vi "Tree Get Node Wild (Usage Mask).vi"(8 "error in (no error)":errorcluster, 9 "Usage mask":i32, 10 "Path":string, 11 "Tree DVR in":refnum<data-value>) -> (0 "error out":errorcluster, 2 "Node array out":refnum<data-value>, 3 "Tree DVR out":refnum<data-value>)   [LabVIEW 2012, in "MDSplus.lvlib"]
doc: "Return the TreeNode array for all the successor nodes of the specified usage with respect of the passed path."
uses:
  <vilib>/MDSplus/Library/MDSplus.lvlib
  <vilib>/MDSplus/Classes/Tree_Class/Tree.lvclass
  <vilib>/MDSplus/Classes/TreeNodeArray_Class/TreeNodeArray.lvclass
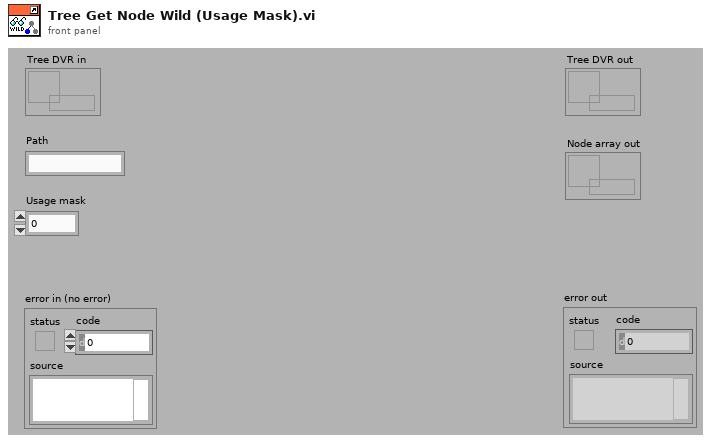
[diagram p1: front panel]
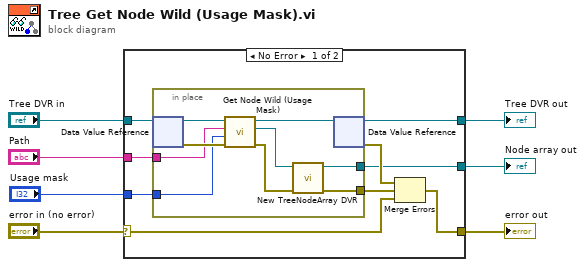
[diagram p0: block diagram]
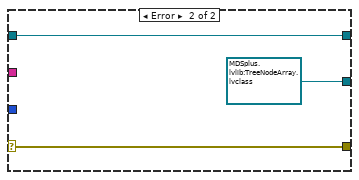
[diagram p2: hidden frame]
diagram:
  n1 = case shown="No Error" "error in (no error)" {
    selector: "error in (no error)" -> [w15 w28]
    tunnel: "Tree DVR in" -> [w16 w27]
    tunnel: [w13 w28] -> w7
    tunnel: [w12 w27] -> w4
    tunnel: [w10 refnum<data-value> refnum ("TreeNode DVR out")] -> w2
    tunnel: "Path" -> [w11 _]
    tunnel: "Usage mask" -> [w8 _]
    frame No Error {
      n2 = in-place {
        in-place-border: [w19] -> w9
        in-place-border: w11 -> [w22]
        in-place-border: [w21] -> w10
        in-place-border: w8 -> [w17]
        n3 = in-place-dvr #1(w16) -> (w25:refnum<class "Tree.lvclass">, w23:errorcluster)
        n4 = call-dynamic "Get Node Wild (Usage Mask).vi"("error in (no error)"=w23, "Usage mask"=w17, "Path"=w22, "Tree in"=w25) -> ("error out"=w20:errorcluster, "Node array out"=w18:refnum<class "TreeNodeArray.lvclass">, "Tree out"=w24:refnum<class "Tree.lvclass">)  [unwired: 5 in]
        n5 = call <vilib>:"New TreeNodeArray DVR.vi"("error in (no error)"=w20, "TreeNodeArray in"=w18) -> ("error out"=w19:errorcluster, "TreeNodeArray DVR out"=w21:refnum<data-value>)  [unwired: 8 in]
        n6 = in-place-dvr #1(w24) -> (w12:refnum<data-value>, w14:errorcluster)
      }
      n7 = Merge Errors(w14, w9, w15) -> (w13:errorcluster)
    }
    frame Error {
    }
  }
  "error out" <- w7
  "Tree DVR out" <- w4
  "Node array out" <- w2
